vi "数据查询_操作日志.vi"() -> ()   [LabVIEW 2016]
uses:
  <vilib>/Utility/miscctls.llb/LVRowAndColumnUnsignedTypeDef.ctl
  <vilib>/Utility/miscctls.llb/LVPointTypeDef.ctl
panel:
  in  "查询":bool
  out "数据表":string[][](table)
  in  "结束日期":string="2020/01/01"
  in  "起始日期":string="2010/01/01"
  in  "组合框":string(combo)
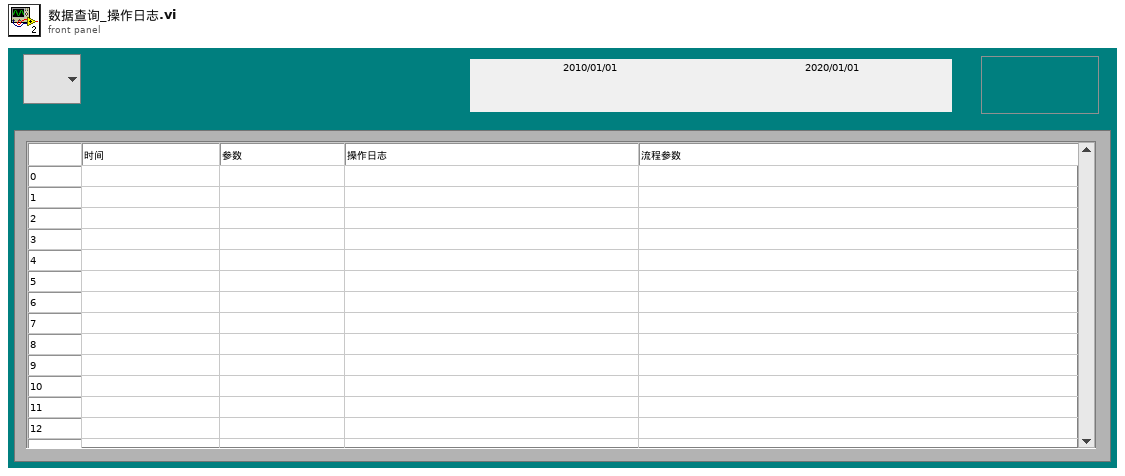
[diagram p1: front panel]
types:
  T1 = typedef "LVRowAndColumnUnsignedTypeDef.ctl" = cluster{"Row":u32, "Column":u32}
  T2 = typedef "LVPointTypeDef.ctl" = cluster{"Horizontal":i16, "Vertical":i16}
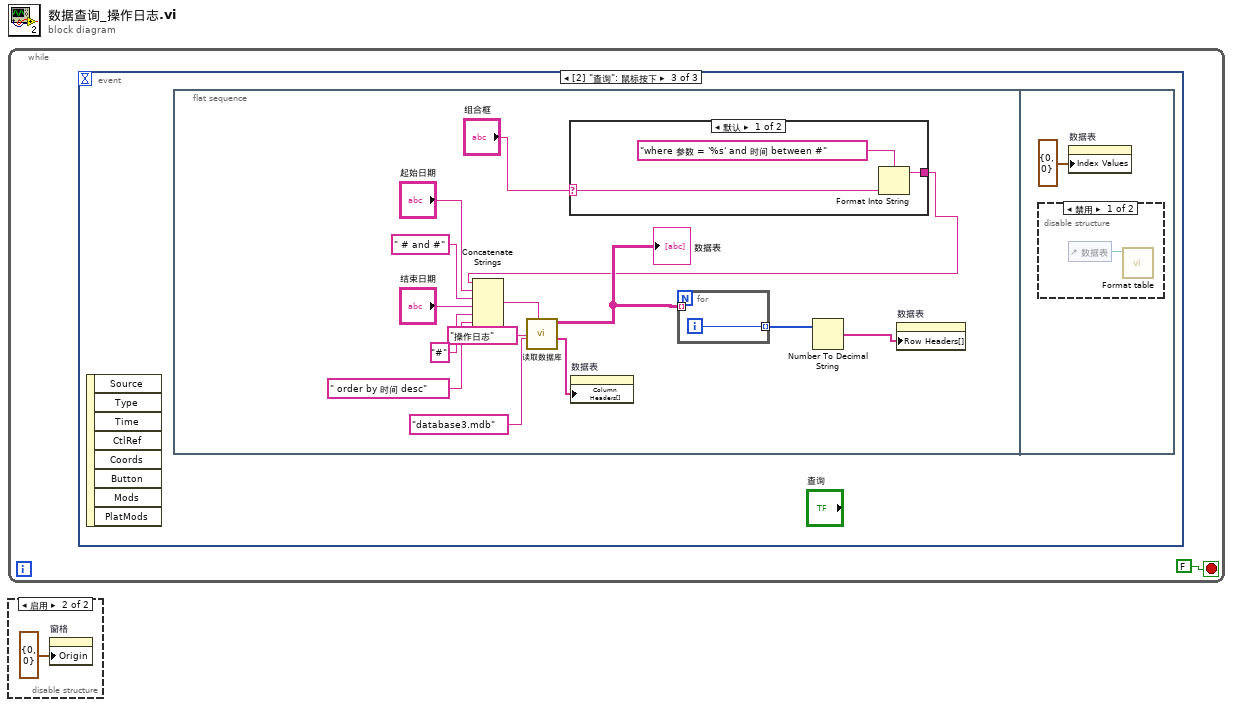
[diagram p0: block diagram]
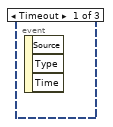
[diagram p2: hidden frame]
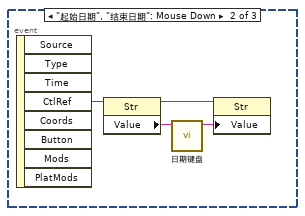
[diagram p3: hidden frame]
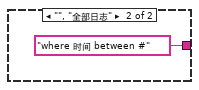
[diagram p4: hidden frame]
diagram:
  n1 = while {
    stop <- FALSE stop-if-true
    n2 = event shown="[2] \"查询\": 鼠标按下" {
      selector: _ -> [_ _ _]
      dyn-events: _ -> [_ _ _]
      timeout: _ -> [_ _ _]
      event Timeout {
        n3 = event-data() -> ()  [unwired: 1 in, 3 out]
      }
      event "起始日期", "结束日期": Mouse Down {
        n4 = event-data() -> ("CtlRef"=w5:refnum<vi>)  [unwired: 1 in, 7 out]
        n5 = property class="Str"(reference=w5) -> (reference out=w3:refnum<vi>, "Value"=w4:string)  [unwired: 1 in, 1 out]
        n6 = call "日期键盘.vi"("原值"=w4) -> ("x+y"=w2:string)  [unwired: 10 in]
        n7 = property class="Str"(reference=w3, "Value"=w2) -> ()  [unwired: 1 in, 2 out]
      }
      event "查询": Mouse Down {
        n8 = event-data() -> ()  [unwired: 1 in, 8 out]
        n9 = flat-sequence {
          frame #0 {
            n10 = case shown="默认" "组合框" {
              selector: "组合框" -> [w20 _]
              tunnel: [w22 "where 时间 between #" ("condition")] -> w6
              frame Default {
                n11 = Format Into String(format string="where 参数 = '%s' and 时间 between #" ("condition"), w20) -> (resulting string=w22:string)  [unwired: 2 in, 1 out]
              }
              frame "", "全部日志" {
              }
            }
            n12 = Concatenate Strings(w6, "起始日期", " # and #" ("condition"), "结束日期", "#" ("condition"), " order by 时间 desc" ("字符串")) -> (w18:string)
            n13 = call "读取数据库.vi"("condition"=w18, "database"="database3.mdb", "组合框"="操作日志") -> ("columns"=w14:string[], "表格"=w11:string[][])  [unwired: 5 in, 2 out]
            "数据表" <- w11
            n14 = property on="数据表" class="Tbl (严格)"("Column Headers[]"=w14) -> ()  [unwired: 2 in, 2 out]
            n15 = for {
              tunnel: w11 -> [_] mode=indexing
              tunnel: [w24] -> w10 mode=indexing
              i -> [w24]
            }
            n16 = Number To Decimal String(number=w10) -> (decimal integer string=w9:string[])  [unwired: 1 in]
            n17 = property on="数据表" class="Tbl (严格)"("Row Headers[]"=w9) -> ()  [unwired: 2 in, 2 out]
          }
          frame #1 {
            n18 = disable-structure shown="禁用" {
              frame Disabled {
                n19 = control-ref of="数据表"() -> (w26:refnum<vi>)
                n20 = call "Format table.vi"("Table输入"=w26) -> ()  [unwired: 11 in]
              }
              frame Enabled {
              }
            }
            n21 = property on="数据表" class="Tbl (严格)"("Index Values"=T1 {"Row"=0, "Column"=0} ("索引值")) -> ()  [unwired: 2 in, 2 out]
          }
        }
      }
    }
  }
  n22 = disable-structure shown="启用" {
    frame Disabled {
    }
    frame Enabled {
      n23 = property on="窗格" class="Pane"("Origin"=T2 {"Horizontal"=0, "Vertical"=0} ("原点")) -> ()  [unwired: 2 in, 2 out]
    }
  }
